vi "Devices Controller_Create.vi"(8 "error in (no error)":errorcluster, 11 "reference in":refnum<class "Devices Controller.lvclass">) -> (0 "error out":errorcluster, 3 "reference out":refnum<class "Devices Controller.lvclass">)   [LabVIEW 2016, in "Devices Controller.lvclass"]
doc: "Constructor."
uses:
  Devices Controller.lvclass
  C:/Program Files (x86)/National Instruments/LabVIEW 2016/vi.lib/addons/_AddQ/G#Object/G#Object.lvclass
  <vilib>/addons/_AddQ/G#Object/G#Object.lvclass
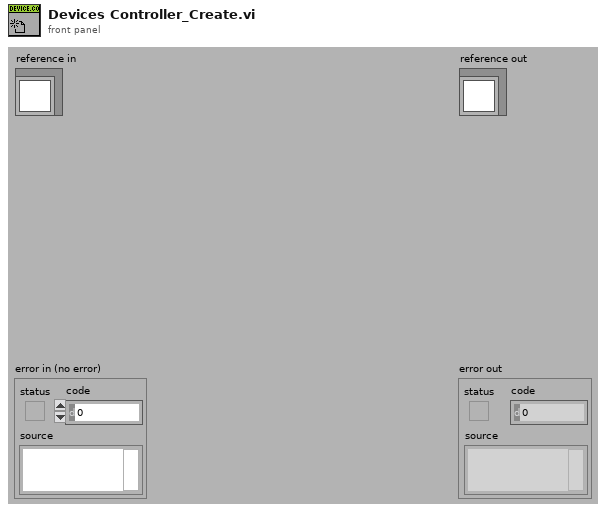
[diagram p1: front panel]
types:
  T1 = typedef "Devices Controller.lvclass/ClassAttributesRef.ctl" = refnum<data-value>
  T2 = typedef "Devices Controller.lvclass/ClassAttributes.ctl" = cluster{"Dummy":bool, "device_controller_ref":refnum<class "Devices Controller.lvclass">}
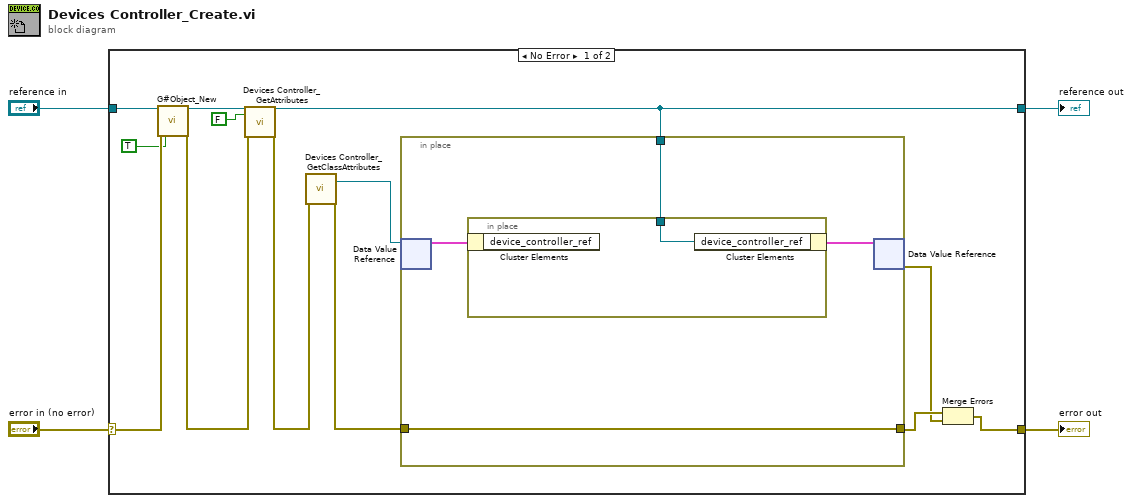
[diagram p0: block diagram]
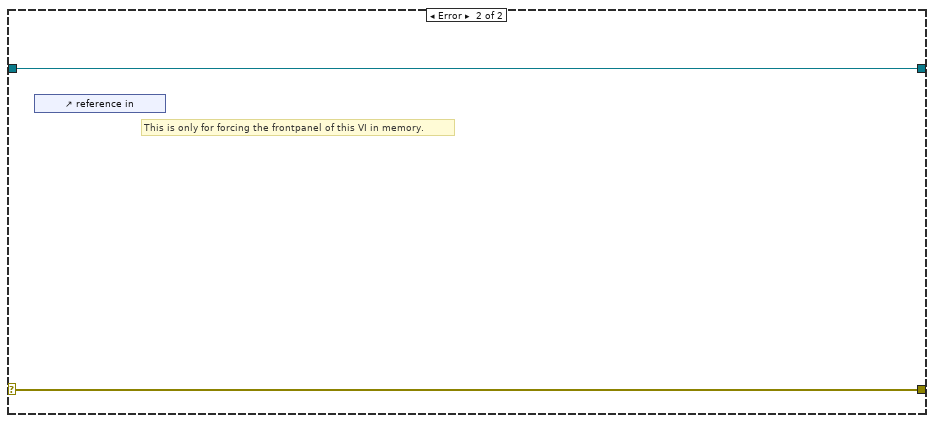
[diagram p2: hidden frame]
diagram:
  n1 = case shown="No Error" "error in (no error)" {
    selector: "error in (no error)" -> [w16 w24]
    tunnel: [w5 w24] -> w3
    tunnel: [w6 w23] -> w1
    tunnel: "reference in" -> [w17 w23]
    frame No Error {
      n2 = call <vilib>:"G#Object_New.vi"("reference in"=w17, "error in (no error)"=w16, "user counter (T)?"=TRUE ("User Counter")) -> ("reference out"=w12:refnum<class "Devices Controller.lvclass">, "error out"=w11:errorcluster)  [unwired: 14 in, 1 out]
      n3 = call "Devices Controller_GetAttributes.vi"("reference in"=w12, "return data? (T)"=FALSE ("return data"), "error in (no error)"=w11) -> ("reference out"=w6:refnum<class "Devices Controller.lvclass">, "error out"=w9:errorcluster)  [unwired: 13 in, 2 out]
      n4 = call "Devices Controller_GetClassAttributes.vi"("error in (no error)"=w9) -> ("class attributes ref"=w7:T1, "error out"=w8:errorcluster)  [unwired: 15 in, 2 out]
      n5 = in-place {
        in-place-border: w8 -> [w19]
        in-place-border: [w19] -> w14
        in-place-border: w6 -> [w18]
        n6 = in-place-dvr #1(w7) -> (w20:T2)  [unwired: 1 out]
        n7 = in-place {
          in-place-border: w18 -> [w22]
          n8 = in-place-cluster #2(w20) -> ()  [unwired: 1 out]
          n9 = in-place-cluster #2("device_controller_ref"=w22) -> (w21:T2)
        }
        n10 = in-place-dvr #1(w21) -> (w13:errorcluster)  [unwired: 1 out]
      }
      n11 = Merge Errors(w14, w13) -> (w5:errorcluster)
    }
    frame Error {
      # "This is only for forcing the frontpanel of this VI in memory."
      n12 = control-ref of="reference in"() -> ()  [unwired: 1 out]
    }
  }
  "error out" <- w3
  "reference out" <- w1
